vi "Flatten repeated.vi"(7 "Field Number":i32, 10 "Data":T1[](array[typedef]) {"Time Stamp" format="%<%x %.3X>T"}, 11 "Buffer in":u8[](array[numeric]) format="%.0x") -> (3 "Buffer":u8[](array[numeric]) format="%.0x")   [LabVIEW 2023, in "ConstellationCommand.lvlib"]
uses:
  ConstellationCommand.lvlib
  <vilib>/IlluminatedG/IG Protoc/LV-Proto/LV-Proto.lvlib
  Data.ctl
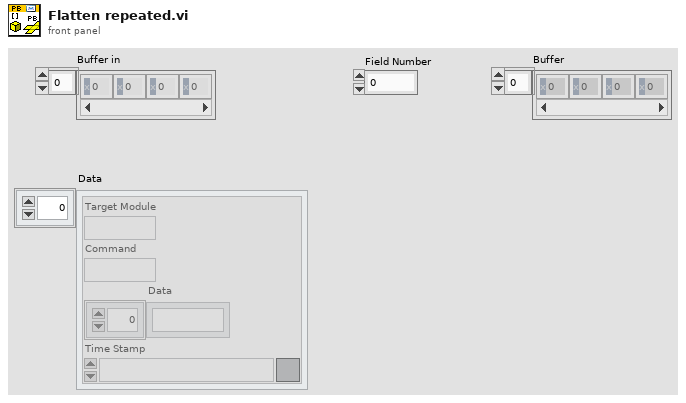
[diagram p1: front panel]
types:
  T1 = typedef "ConstellationCommand.lvlib/Data.ctl" = cluster{"Target Module":string, "Command":string, "Data":string[], "Time Stamp":timestamp}
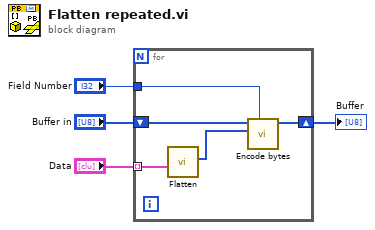
[diagram p0: block diagram]
diagram:
  n1 = for {
    tunnel: "Field Number" -> [w8]
    shift-right: [w7] -> w2
    shift-left: "Buffer in" -> [w9]
    tunnel: "Data" -> [w6] mode=indexing
    n2 = call "Flatten.vi"("Command Data"=w6) -> ("Buffer"=w5:u8[])  [unwired: 9 in, 1 out]
    n3 = call <vilib>:"Encode bytes.vi"("Field Number"=w8, "bytes"=w5, "Buffer in"=w9) -> ("Buffer"=w7:u8[])  [unwired: 8 in]
  }
  "Buffer" <- w2
